vi "AOC1_Part2.vi"() -> ()   [LabVIEW 2015]
panel:
  out "Character Position":i32
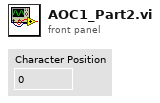
[diagram p1: front panel]
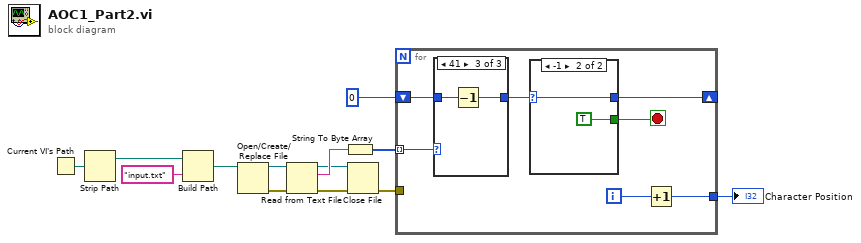
[diagram p0: block diagram]
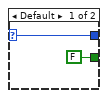
[diagram p2: hidden frame]
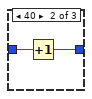
[diagram p4: hidden frame]
diagram:
  n1 = Current VI's Path() -> (path=w11:path)
  n2 = Strip Path(path=w11) -> (stripped path=w10:path)  [unwired: 1 out]
  n3 = Build Path(base path=w10, name or relative path="input.txt") -> (appended path=w8:path)
  n4 = Open/Create/Replace File(file path (use dialog)=w8) -> (refnum out=w12:refnum<file>, error out=w13:errorcluster)  [unwired: 5 in, 1 out]
  n5 = Read from Text File(file (use dialog)=w12, error in=w13) -> (refnum out=w5:refnum<file>, text=w7:string, error out=w6:errorcluster)  [unwired: 2 in, 1 out]
  n6 = String To Byte Array(string=w7) -> (unsigned byte array=w4:u8[])
  n7 = Close File(refnum=w5, error in=w6) -> (error out=w3:errorcluster)  [unwired: 1 out]
  n8 = for {
    tunnel: w4 -> [w20] mode=indexing
    tunnel: w3 -> [_]
    shift-right: [w17] -> _
    shift-left: 0 -> [w19]
    tunnel: [w14] -> w1
    i -> [w15]
    stop <- w16 stop-if-true
    n9 = case shown="41" w20 {
      tunnel: w19 -> [w25 w27 w29]
      tunnel: [w25 w26 w28] -> w18
      frame Default {
      }
      frame 40 {
        n10 = Increment(x=w27) -> (x+1=w26:i32)
      }
      frame 41 {
        n11 = Decrement(x=w29) -> (x-1=w28:i32)
      }
    }
    n12 = case shown="-1" w18 {
      selector: w18 -> [w22 w24]
      tunnel: [w22 w24] -> w17
      tunnel: [FALSE TRUE] -> w16
      frame Default {
      }
      frame -1 {
      }
    }
    n13 = Increment(x=w15) -> (x+1=w14:i32)
  }
  "Character Position" <- w1
